vi "ImagePathAndSavePathToDatabase(SubVI).vi"(0 "connection reference":T1, 1 "Name":string, 2 "QuestionsNo_Ordered":string) -> (5 "ImagePath":path)   [LabVIEW 2013]
uses:
  <vilib>/addons/database/Connection.llb/Conn ObjectReference.ctl
  <vilib>/Utility/sysdir.llb/System Directory Type.ctl
  FYP_LabviewGlobal(SubVI).vi
  <vilib>/addons/database/NI_Database_API.lvlib
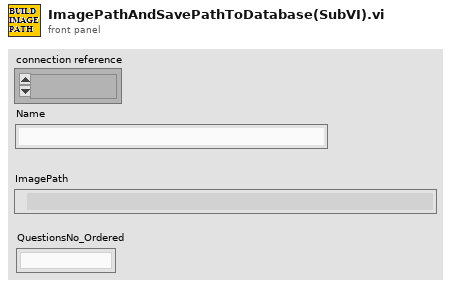
[diagram p1: front panel]
types:
  T1 = typedef "NI_Database_API.lvlib/Conn ObjectReference.ctl" = refnum<k1>
  T2 = typedef "System Directory Type.ctl" = i32
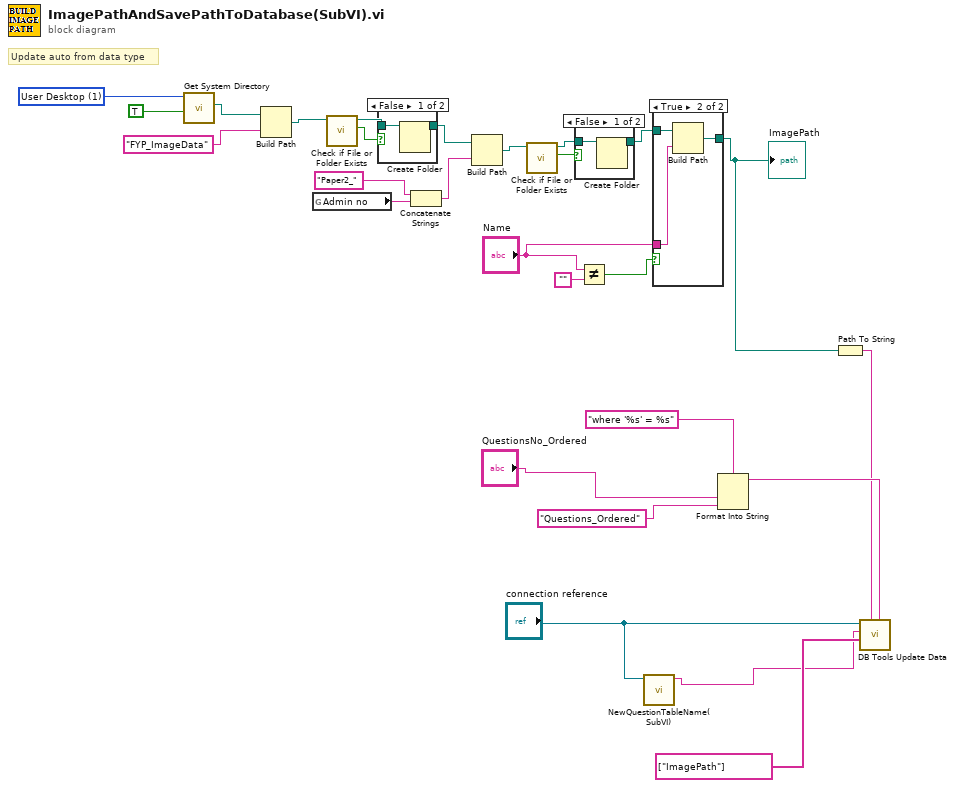
[diagram p0: block diagram]
diagram:
  w27 = T2 1 items=["User Home"=0, "User Desktop"=1, "User Documents"=2, "User Application Data"=3, "User Preferences"=4, "User Temporary"=5, "Public Documents"=6, "Public Application Data"=7, "Public Preferences"=8, "Public Cache"=13, "System Core Libraries"=9, "System Installed Libraries"=10, "Application Files"=11, "Boot Volume Root"=12] ("system directory type")
  # "Update auto from data type"
  n1 = call <vilib>:"Get System Directory.vi"("create directory if not found? (F)"=TRUE, "system directory type"=w27) -> ("system directory"=w25:path)  [unwired: 9 in]
  n2 = Build Path(base path=w25, name or relative path="FYP_ImageData") -> (appended path=w23:path)
  n3 = global read "FYP_LabviewGlobal(SubVI).vi" "Admin no"() -> (w12:string)
  n4 = call <vilib>:"Check if File or Folder Exists.vi"("path"=w23) -> ("file or folder exists?"=w21:bool, "dup path"=w22:path)  [unwired: 8 in, 1 out]
  n5 = case shown="False" w21 {
    tunnel: w22 -> [w29 w30]
    tunnel: [w28 w30] -> w16
    frame False {
      n6 = Create Folder(path (use dialog)=w29) -> (created path=w28:path)  [unwired: 2 in, 2 out]
    }
    frame True {
    }
  }
  n7 = Concatenate Strings("Paper2_", w12) -> (w10:string)
  n8 = Build Path(base path=w16, name or relative path=w10) -> (appended path=w17:path)
  n9 = call <vilib>:"Check if File or Folder Exists.vi"("path"=w17) -> ("file or folder exists?"=w14:bool, "dup path"=w15:path)  [unwired: 8 in, 1 out]
  n10 = case shown="False" w14 {
    tunnel: w15 -> [w32 w33]
    tunnel: [w31 w33] -> w13
    frame False {
      n11 = Create Folder(path (use dialog)=w32) -> (created path=w31:path)  [unwired: 2 in, 2 out]
    }
    frame True {
    }
  }
  n12 = Not Equal?(x="Name", y="") -> (x != y?=w18:bool)
  n13 = call "NewQuestionTableName(SubVI).vi"("connection reference"="connection reference") -> ("String"=w2:string)  [unwired: 9 in, 1 out]
  n14 = case shown="True" w18 {
    tunnel: [w34 w37] -> w3
    tunnel: w13 -> [w34 w36]
    tunnel: "Name" -> [_ w35]
    frame False {
    }
    frame True {
      n15 = Build Path(base path=w36, name or relative path=w35) -> (appended path=w37:path)
    }
  }
  "ImagePath" <- w3
  n16 = Format Into String(format string="where '%s' = %s", "QuestionsNo_Ordered", "Questions_Ordered") -> (resulting string=w5:string)  [unwired: 2 in, 1 out]
  n17 = Path To String(path=w3) -> (string=w4:string)
  n18 = call <vilib>:"DB Tools Update Data.vi"("condition"=w5, "data"=w4, "columns"=string[] ["ImagePath"], "table"=w2, "connection reference"="connection reference") -> ()  [unwired: 5 in, 2 out]
